vi "get record playback values.vi"(9 "Track Enable":T3, 10 "Audio In":T2, 11 "4-Track Audio in":T1) -> (3 "4-Track Audio out":T1)   [LabVIEW 2014]
uses:
  Controls/Audio In.ctl
  Controls/4 Track Audio.ctl
  Controls/Track Enable.ctl
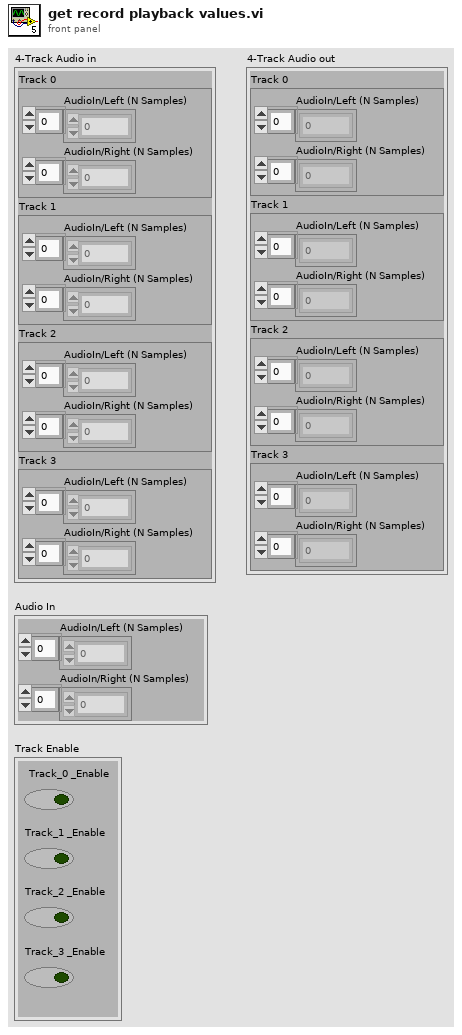
[diagram p1: front panel]
types:
  T1 = typedef "4 Track Audio.ctl" = cluster{"Track 0":T2, "Track 1":T2, "Track 2":T2, "Track 3":T2}
  T2 = typedef "Audio In.ctl" = cluster{"AudioIn/Left (N Samples)":i16[], "AudioIn/Right (N Samples)":i16[]}
  T3 = typedef "Track Enable.ctl" = cluster{"Track_0 _Enable ":bool, "Track_1 _Enable ":bool, "Track_2 _Enable ":bool, "Track_3 _Enable ":bool}
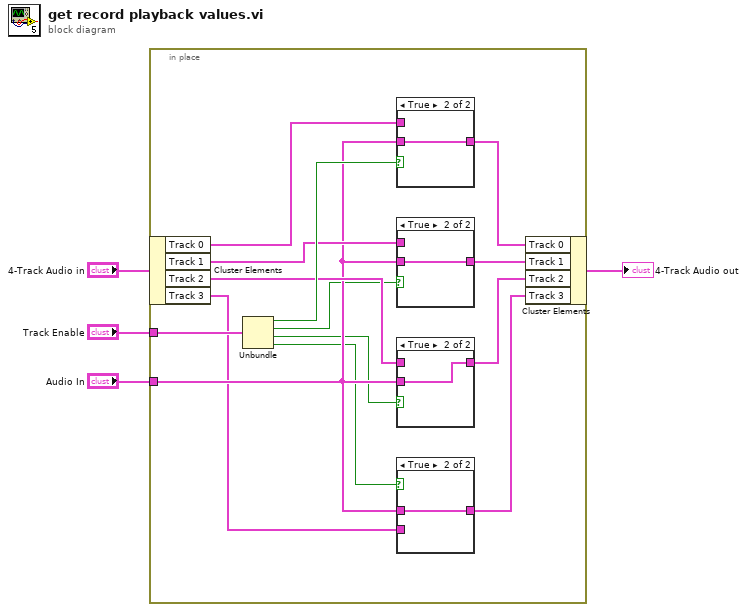
[diagram p0: block diagram]
diagram:
  n1 = in-place {
    in-place-border: "Track Enable" -> [w18]
    in-place-border: "Audio In" -> [w12]
    n2 = in-place-cluster #1("4-Track Audio in") -> ("Track 0"=w16:T2, "Track 1"=w14:T2, "Track 2"=w13:T2, "Track 3"=w11:T2)
    n3 = Unbundle(w18) -> ("Track_0 _Enable"=w17:bool, "Track_1 _Enable"=w7:bool, "Track_2 _Enable"=w6:bool, "Track_3 _Enable"=w5:bool)
    n4 = case shown="True" w17 {
      tunnel: w16 -> [w25 _]
      tunnel: [w25 w26] -> w15
      tunnel: w12 -> [_ w26]
      frame False {
      }
      frame True {
      }
    }
    n5 = case shown="True" w7 {
      tunnel: w14 -> [w23 _]
      tunnel: [w23 w24] -> w10
      tunnel: w12 -> [_ w24]
      frame False {
      }
      frame True {
      }
    }
    n6 = case shown="True" w6 {
      tunnel: w13 -> [w21 _]
      tunnel: [w21 w22] -> w9
      tunnel: w12 -> [_ w22]
      frame False {
      }
      frame True {
      }
    }
    n7 = case shown="True" w5 {
      tunnel: w11 -> [w19 _]
      tunnel: [w19 w20] -> w8
      tunnel: w12 -> [_ w20]
      frame False {
      }
      frame True {
      }
    }
    n8 = in-place-cluster #1("Track 0"=w15, "Track 1"=w10, "Track 2"=w9, "Track 3"=w8) -> (→"4-Track Audio out":T1)
  }
